vi "ModifyClassAttribute1.vi"(1 "Lock time (ms)":u32, 5 "error in (no error)":errorcluster) -> (19 "error out":errorcluster)   [LabVIEW 2017, in "G#SubClass1.lvclass"]
uses:
  G#SubClass1.lvclass
  G#BaseClass1_class/G#BaseClass1.lvclass
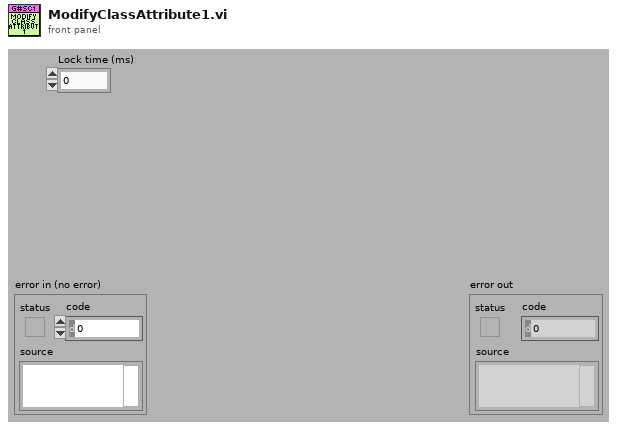
[diagram p1: front panel]
types:
  T1 = typedef "G#BaseClass1.lvclass/ClassAttributesRef.ctl" = refnum<data-value>
  T2 = typedef "G#SubClass1.lvclass/ClassAttributesRef.ctl" = refnum<data-value>
  T3 = typedef "G#SubClass1.lvclass/ClassAttributes.ctl" = cluster{"SubClassIntAttribute":i32}
  T4 = typedef "G#BaseClass1.lvclass/ClassAttributes.ctl" = cluster{"Int":i32, "ArrayInt":i32[]}
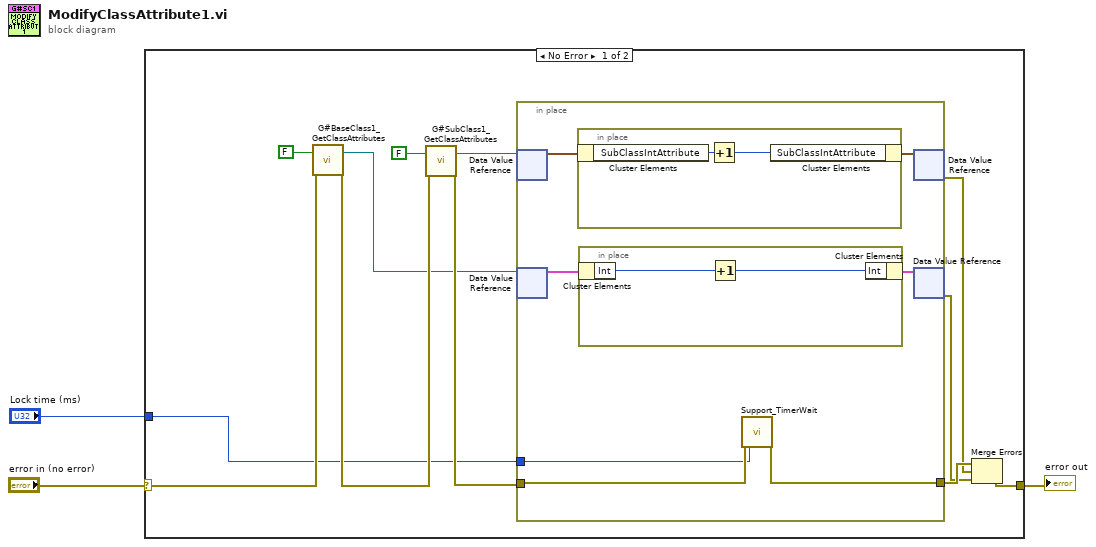
[diagram p0: block diagram]
diagram:
  n1 = case shown="No Error" "error in (no error)" {
    selector: "error in (no error)" -> [w9 w27]
    tunnel: [w13 w27] -> w2
    tunnel: "Lock time (ms)" -> [w4 _]
    frame No Error {
      n2 = call "G#BaseClass1_GetClassAttributes.vi"("return data? (T)"=FALSE ("return data"), "error in (no error)"=w9) -> ("class attributes ref"=w6:T1, "error out"=w8:errorcluster)  [unwired: 14 in, 2 out]
      n3 = call "G#SubClass1_GetClassAttributes.vi"("return data? (T)"=FALSE ("return data"), "error in (no error)"=w8) -> ("class attributes ref"=w14:T2, "error out"=w15:errorcluster)  [unwired: 14 in, 2 out]
      n4 = in-place {
        in-place-border: w15 -> [w18]
        in-place-border: [w17] -> w11
        in-place-border: w4 -> [w16]
        n5 = in-place-dvr #1(w14) -> (w21:T3)  [unwired: 1 out]
        n6 = in-place-dvr #2(w6) -> (w20:T4)  [unwired: 1 out]
        n7 = in-place {
          n8 = in-place-cluster #3(w21) -> ("SubClassIntAttribute"=w26:i32)
          n9 = Increment(x=w26) -> (x+1=w25:i32)
          n10 = in-place-cluster #3("SubClassIntAttribute"=w25) -> (w22:T3)
        }
        n11 = in-place {
          n12 = in-place-cluster #4(w20) -> ("Int"=w24:i32)
          n13 = Increment(x=w24) -> (x+1=w23:i32)
          n14 = in-place-cluster #4("Int"=w23) -> (w19:T4)
        }
        n15 = call "Support_TimerWait.vi"("error in (no error)"=w18, "milliseconds to wait"=w16) -> ("error out"=w17:errorcluster)  [unwired: 17 in]
        n16 = in-place-dvr #1(w22) -> (w10:errorcluster)  [unwired: 1 out]
        n17 = in-place-dvr #2(w19) -> (w5:errorcluster)  [unwired: 1 out]
      }
      n18 = Merge Errors(w11, w10, w5) -> (w13:errorcluster)
    }
    frame Error {
    }
  }
  "error out" <- w2
